vi "5.6.vi"() -> ()   [LabVIEW 2017]
uses:
  <vilib>/measure/NI_MABase.lvlib
panel:
  out "最大值":dbl
  out "大小":i32
  out "dt":dbl
  out "Y":dbl[](array[numeric])
  in  "sampling info":cluster{"Fs":dbl, "#s":dbl}={"Fs"=1000.0, "#s"=1000.0} caption="采样信息" {"Fs" format="%.2p"}
  in  "phase":dbl caption="相位" format="%.2p"
  in  "amplitude":dbl=1.0 caption="幅值" format="%0.2p"
  in  "frequency":dbl=10.0 caption="频率" format="%0.2p"
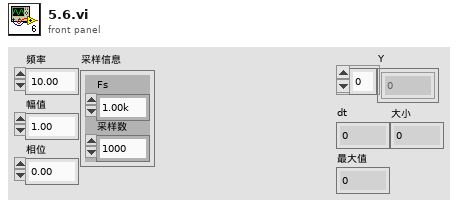
[diagram p1: front panel]
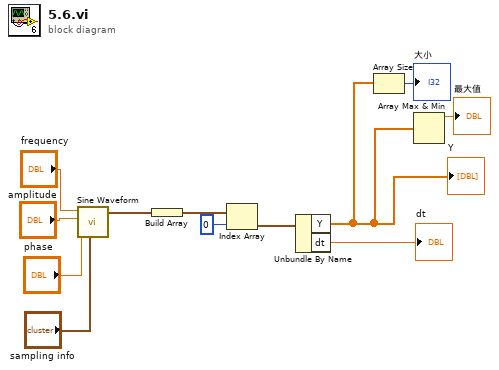
[diagram p0: block diagram]
diagram:
  n1 = call <vilib>:"Sine Waveform.vi"("sampling info"="sampling info", "phase"="phase", "amplitude"="amplitude", "frequency"="frequency") -> ("signal out"=w8:waveform(dbl))  [unwired: 6 in, 1 out]
  n2 = Build Array(w8) -> (w7:waveform(dbl)[])
  n3 = Index Array(array=w7, index=0) -> (element=w5:waveform(dbl))
  n4 = Unbundle By Name(w5) -> ("Y"=w2:dbl[], "dt"=→"dt":dbl)
  "Y" <- w2
  n5 = Array Size(array=w2) -> (size(s)=→"大小":i32)
  n6 = Array Max & Min(array=w2) -> (max value=→"最大值":dbl)  [unwired: 3 out]
